vi "Move Item in Listbox.vi"(7 "Move All Items? (f)":bool, 10 "Destination Lisbox":refnum<vi>, 11 "Source Listbox":refnum<vi>) -> ()   [LabVIEW 2017]
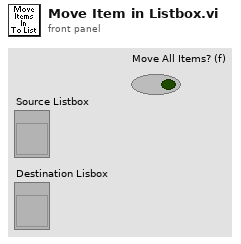
[diagram p1: front panel]
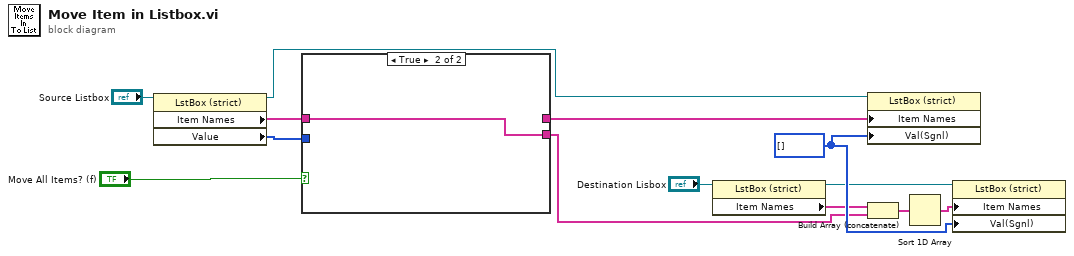
[diagram p0: block diagram]
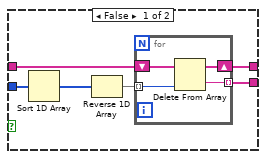
[diagram p2: hidden frame]
diagram:
  w13 = i32[] [] ("Actors")
  n1 = property on="Property Node" class="LstBox (strict)"(reference="Source Listbox") -> (reference out=w5:refnum<vi>, "Item Names"=w8:string[], "Value"=w9:i32[])  [unwired: 1 in, 1 out]
  n2 = case shown="True" "Move All Items? (f)" {
    tunnel: [w19 w24] -> w1
    tunnel: [w18 _] -> w10
    tunnel: w9 -> [w15 _]
    tunnel: w8 -> [w14 w24]
    frame False {
      n3 = Sort 1D Array(array=w15) -> (sorted array=w17:i32[])
      n4 = Reverse 1D Array(array=w17) -> (reversed array=w16:i32[])
      n5 = for {
        tunnel: w16 -> [w22] mode=indexing
        shift-right: [w21] -> w18
        shift-left: w14 -> [w23]
        tunnel: [w20] -> w19 mode=indexing
        n6 = Delete From Array(array=w23, index=w22) -> (deleted portion=w20:string, array with subset deleted=w21:string[])  [unwired: 1 in]
      }
    }
    frame True {
    }
  }
  n7 = property on="Property Node" class="LstBox (strict)"(reference="Destination Lisbox") -> (reference out=w3:refnum<vi>, "Item Names"=w2:string[])  [unwired: 1 in, 1 out]
  n8 = property on="Property Node" class="LstBox (strict)"(reference=w5, "Item Names"=w10, "Val(Sgnl)"=w13) -> ()  [unwired: 1 in, 2 out]
  n9 = Build Array (concatenate)(w2, w1) -> (w11:string[])
  n10 = Sort 1D Array(array=w11) -> (sorted array=w12:string[])
  n11 = property on="Property Node" class="LstBox (strict)"(reference=w3, "Item Names"=w12, "Val(Sgnl)"=w13) -> ()  [unwired: 1 in, 2 out]
